vi "scaleEncoders.vi"(8 "error in (no error)":errorcluster, 11 "String":string) -> (0 "error out":errorcluster, 2 "Encoder1":u32, 3 "Encoder0":u32)   [LabVIEW 2017, in "externalAquisition.lvlib"]
doc: "This VI scales the string into an encoder count"
uses:
  externalAquisition.lvlib
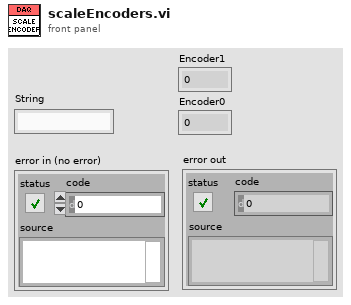
[diagram p1: front panel]
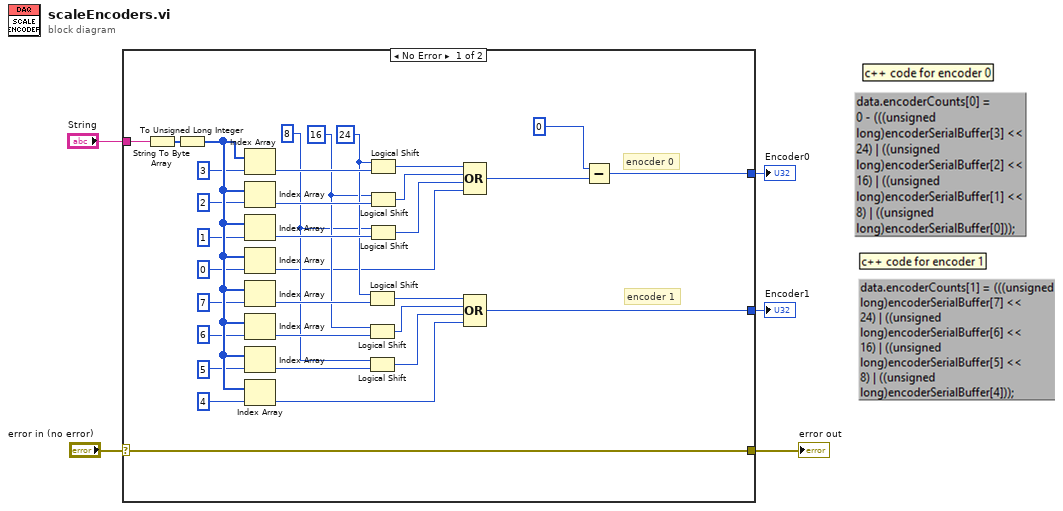
[diagram p0: block diagram]
diagram:
  n1 = case shown="No Error" "error in (no error)" {
    selector: "error in (no error)" -> [w27 w39]
    tunnel: "String" -> [w38 _]
    tunnel: [w27 w39] -> w3
    tunnel: [w9 _] -> w2
    tunnel: [w6 _] -> w1
    frame No Error {
      w18 = 8
      w19 = 16
      w20 = 24
      # "encoder 1"
      # "enocder 0"
      n2 = String To Byte Array(string=w38) -> (unsigned byte array=w37:u8[])
      n3 = To Unsigned Long Integer(number=w37) -> (unsigned 32bit integer=w36:u32[])
      n4 = Index Array(array=w36, index=3) -> (element=w26:u32)
      n5 = Index Array(array=w36, index=2) -> (element=w25:u32)
      n6 = Index Array(array=w36, index=1) -> (element=w24:u32)
      n7 = Index Array(array=w36, index=0) -> (element=w14:u32)
      n8 = Index Array(array=w36, index=7) -> (element=w23:u32)
      n9 = Index Array(array=w36, index=6) -> (element=w22:u32)
      n10 = Index Array(array=w36, index=5) -> (element=w21:u32)
      n11 = Index Array(array=w36, index=4) -> (element=w10:u32)
      n12 = Logical Shift(y=w20, x=w23) -> (x << y=w13:u32)
      n13 = Logical Shift(y=w19, x=w22) -> (x << y=w12:u32)
      n14 = Logical Shift(y=w18, x=w21) -> (x << y=w11:u32)
      n15 = Logical Shift(y=w20, x=w26) -> (x << y=w17:u32)
      n16 = Logical Shift(y=w19, x=w25) -> (x << y=w16:u32)
      n17 = Logical Shift(y=w18, x=w24) -> (x << y=w15:u32)
      n18 = Compound Arithmetic op=OR(w17, w16, w15, w14) -> (w7:u32)
      n19 = Compound Arithmetic op=OR(w13, w12, w11, w10) -> (w9:u32)
      n20 = Subtract(x=u32 0, y=w7) -> (x-y=w6:u32)
    }
    frame Error {
    }
  }
  "error out" <- w3
  "Encoder1" <- w2
  "Encoder0" <- w1
